vi "Name.vi"(8 "error in (no error)":errorcluster, 11 "LUnit Test Case in":refnum<class "LUnit Test Case.lvclass">) -> (0 "error out":errorcluster, 2 "Name":string, 3 "LUnit Test Case out":refnum<class "LUnit Test Case.lvclass">)   [LabVIEW 2020, in "LUnit Test Case.lvclass"]
doc: "Returns name of test."
uses:
  LUnit Test Case.lvclass
  LUnit Test Case.lvclass/LUnit Test Case.ctl
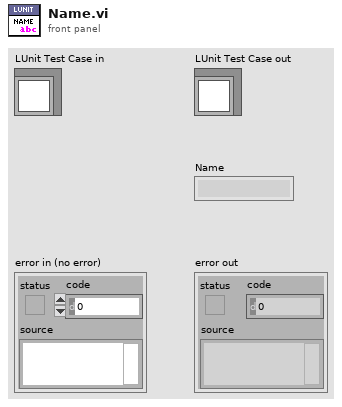
[diagram p1: front panel]
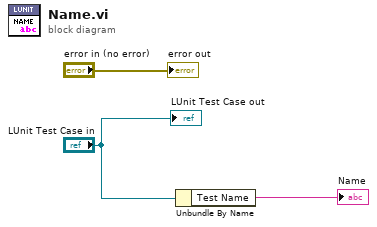
[diagram p0: block diagram]
diagram:
  n1 = Unbundle By Name("LUnit Test Case in") -> ("Test Name"=→"Name":string)
  "error out" <- "error in (no error)"
  "LUnit Test Case out" <- "LUnit Test Case in"
